vi "FTW-Endpoint-Receive.vi"(0 "FTW Endpoint":refnum<class "FTW-Endpoint-Notifier.lvclass">, 5 "Timeout":i32 format="%dmsec", 11 "error in":errorcluster) -> (4 "FTW Endpoint out":refnum<class "FTW-Endpoint-Notifier.lvclass">, 6 "Message Header":string, 8 "Message Body":string, 10 "Timed out?":bool, 15 "error out":errorcluster)   [LabVIEW 2012, in "FTW-Actor.lvlib" / "FTW-Endpoint-Notifier.lvclass"]
uses:
  FTW-Endpoint-Notifier.lvclass
  FTW-Endpoint-Notifier.lvclass/FTW-Endpoint-Notifier.ctl
panel:
  # "Inputs"
  # "Outputs"
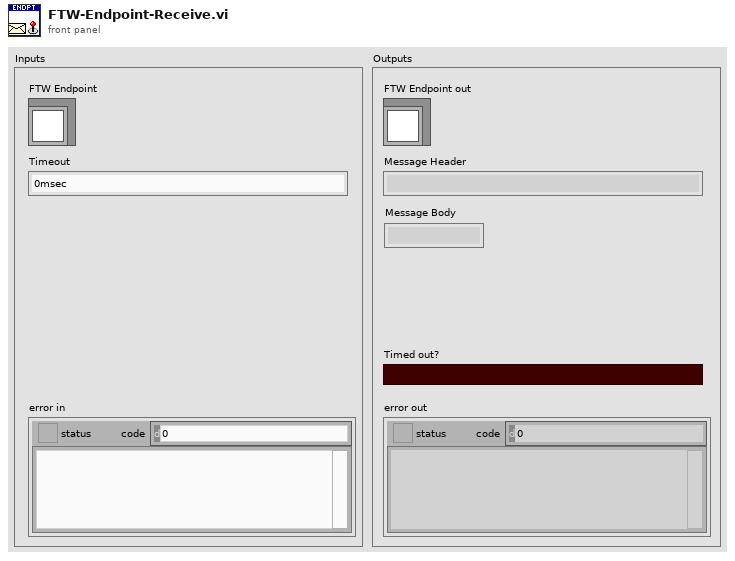
[diagram p1: front panel]
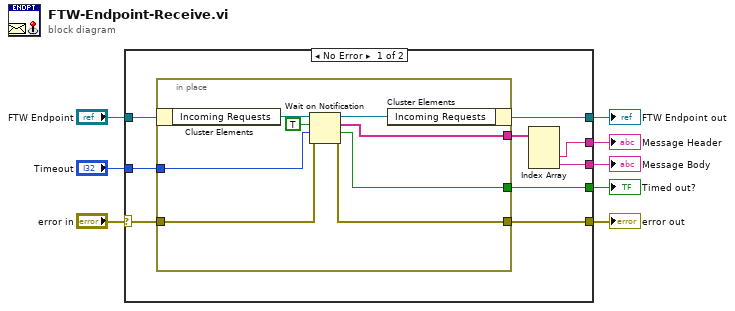
[diagram p0: block diagram]
diagram:
  n1 = case shown="No Error" "error in" {
    selector: "error in" -> [w11 w27]
    tunnel: [w10 w27] -> w8
    tunnel: [w14 w26] -> w6
    tunnel: "FTW Endpoint" -> [w15 w26]
    tunnel: [w9 _] -> w4
    tunnel: "Timeout" -> [w12 _]
    tunnel: [w17 _] -> w2
    tunnel: [w16 _] -> w1
    frame No Error {
      n2 = in-place {
        in-place-border: [w22] -> w10
        in-place-border: w11 -> [w23]
        in-place-border: w12 -> [w24]
        in-place-border: [w20] -> w13
        in-place-border: [w19] -> w9
        n3 = in-place-cluster #1(w15) -> ("Incoming Requests"=w25:refnum<notifier>)
        n4 = Wait on Notification(notifier=w25, ignore previous (F)=TRUE, timeout in ms (-1)=w24, error in (no error)=w23) -> (notifier out=w21:refnum<notifier>, notification=w20:string[], timed out?=w19:bool, error out=w22:errorcluster)
        n5 = in-place-cluster #1("Incoming Requests"=w21) -> (w14:refnum<class "FTW-Endpoint-Notifier.lvclass">)
      }
      n6 = Index Array(array=w13) -> (element #2=w17:string, element #3=w16:string)  [unwired: 3 in, 1 out]
    }
    frame Error {
    }
  }
  "error out" <- w8
  "FTW Endpoint out" <- w6
  "Timed out?" <- w4
  "Message Header" <- w2
  "Message Body" <- w1
